vi "API - Handle Error.vi"(8 "Error In":errorcluster, 11 "Show Error Window?":T1) -> (0 "Error Out":errorcluster)   [LabVIEW 2016, in "Error Manager.lvlib"]
doc: "This VI\n1. If \"Error In\" contains no error this VI does nothing.\n2. If \"Error In\" contains an error:\n 2.1. Sends (enqueues) the error to the Error Manager asynchronous module. That module will \"handle\" the error, i.e. log the error to a file, and (optionally) pop-up an error message to the user.\n 2.2. Clears the error such that the calling VI is guaranteed to \"get rid\" of the error. Such that the caller VI can continue operating because the error was cleared.\n\nNote: This VI guarantees that \"Error Out\" will always contain \"No Error\". There is no need to use a \"Clear Errors\" VI immediately after this VI."
uses:
  Error Manager.lvlib
  Private VIs/Reported Error (cluster).ctl
  Queues/MHL Queue/MHL Queue.lvclass
  Queues/MHL Queue/Command (enum).ctl
  Show Error Window Instruction (enum).ctl
panel:
  # "Input\nInputs to the VI"
  # "Development\nControls or indicators that are useful for development or testing, but which are not outputs of the VI."
  # "Output\nOutputs of the VI"
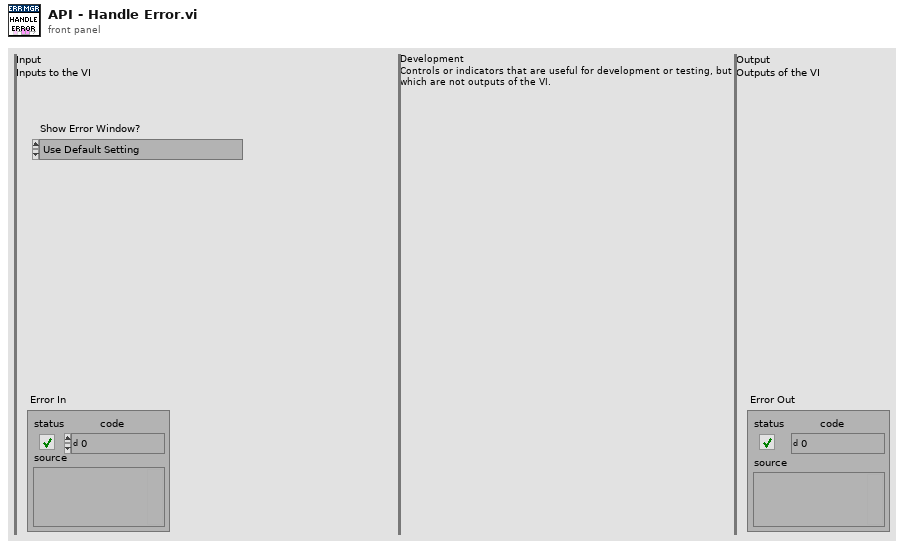
[diagram p1: front panel]
types:
  T1 = typedef "Error Manager.lvlib/Show Error Window Instruction (enum).ctl" = enum16{"Use Default Setting", "Show", "Do Not Show"}
  T2 = typedef "Error Manager.lvlib/MHL Queue.lvclass/Command (enum).ctl" = enum16{"Init Module", "Close Module", "Internal Error", "Create Error Log File", "Show Front Panel", "Handle Error", "Refresh MCL", "MCL Value Change", "Change Display Order", "One-Second Interval Expired", "Mark Selected Errors As Read", "Mark All Errors As Read", "Refresh Button State - MSEAR", "Refresh Button State - MAEAR"}
  T3 = typedef "Error Manager.lvlib/Reported Error (cluster).ctl" = cluster{"Error Timestamp":timestamp, "Error Code":i32, "Error message":string, "Show Error Window?":T1}
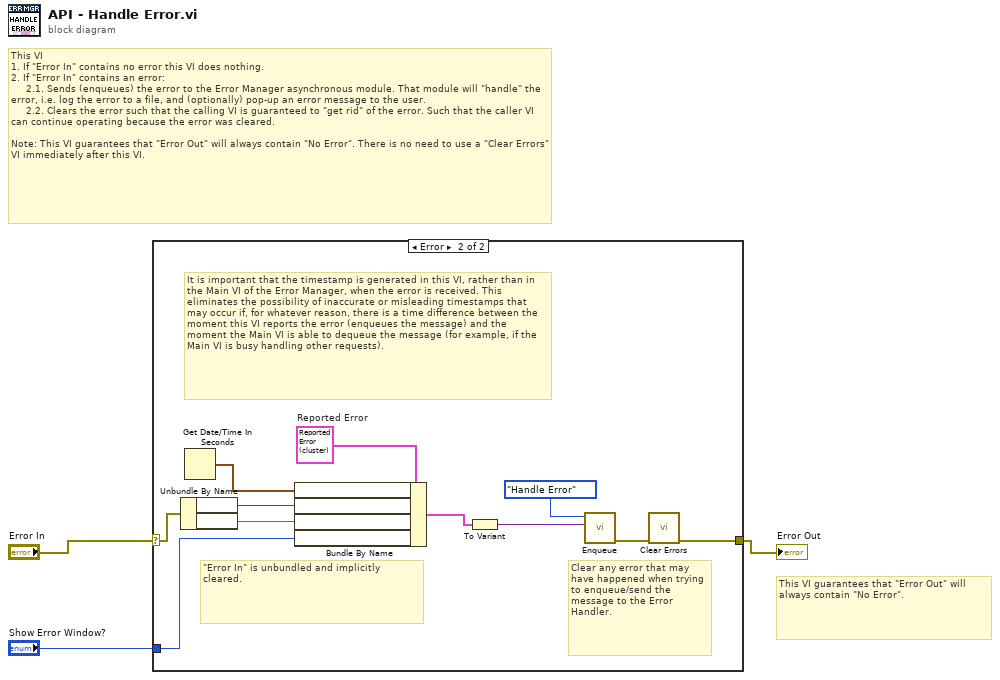
[diagram p0: block diagram]
diagram:
  # "This VI guarantees that \"Error Out\" will always contain \"No Error\"."
  # "This VI\n1. If \"Error In\" contains no error this VI does nothing.\n2. If \"Error In\" contains an error:\n     2.1. Sends (enqueues) the error to the Error Manager asynchronous module. That module will \"handle\" the error, i.e. log the error to a file, and (optionally) pop-up an error message to the user.\n     2.2. Clears the error such that the calling VI is guaranteed to \"get rid\" of the error. Such that the caller VI can continue operating because the error was cleared.\n\nNote: This VI guarantees that \"Error Out\" will always contain \"No Error\". There is no need to use a \"Clear Errors\" VI immediately after this VI."
  n1 = case shown="Error" "Error In" {
    selector: "Error In" -> [w4 w10]
    tunnel: [w4 w13] -> w2
    tunnel: "Show Error Window?" -> [_ w5]
    frame No Error {
    }
    frame Error {
      w12 = T3 {"Error Timestamp"=timestamp(0 s since 1904-01-01), "Error Code"=0, "Error message"="", "Show Error Window?"=enum."Use Default Setting"}  # Reported Error
      # "It is important that the timestamp is generated in this VI, rather than in the Main VI of the Error Manager, when the error is received. This eliminates the possibility of inaccurate or misleading timestamps that may occur if, for whatever reason, there is a time difference between the moment this VI reports the error (enqueues the message) and the moment the Main VI is able to dequeue the message (for example, if the Main VI is busy handling other requests)."
      # "Clear any error that may have happened when trying to enqueue/send the message to the Error Handler."
      # "\"Error In\" is unbundled and implicitly cleared."
      n2 = Unbundle By Name(w10) -> (w9:i32, w7:string)
      n3 = Get Date/Time In Seconds() -> (seconds since 1Jan1904=w8:timestamp)
      n4 = Bundle By Name(cluster=w12, w8, w9, w7, w5) -> (w11:T3)
      n5 = To Variant(anything=w11) -> (Variant=w15:variant)
      n6 = call "Enqueue.vi"(10:w15, 11:Command_(enum)."Handle Error" ("Command")) -> (0:w14:errorcluster)  [unwired: 9 in]
      n7 = call <vilib>:"Clear Errors.vi"(4:w14) -> (0:w13:errorcluster)  [unwired: 5 in, 1 out]
    }
  }
  "Error Out" <- w2
